vi "Process Mouse Up.vi"(0 "Listbox":refnum<vi>, 1 "Ring":refnum<vi>, 5 "State in":T1, 7 "Coords":T6, 11 "error in (no error)":errorcluster) -> (6 "State out":T1, 8 "state changed":bool, 15 "error out":errorcluster)   [LabVIEW 2020, in "KTable.xctl"]
uses:
  KTable.xctl
  <vilib>/Utility/miscctls.llb/LVPoint32TypeDef.ctl
  State.ctl
  ColumnSpec.ctl
  ColumnType.ctl
  Table Properties.ctl
  Events.ctl
  Event Data.ctl
  Event Type.ctl
  Array Manipulation VIs/Array-Dimensions (2D string).vi
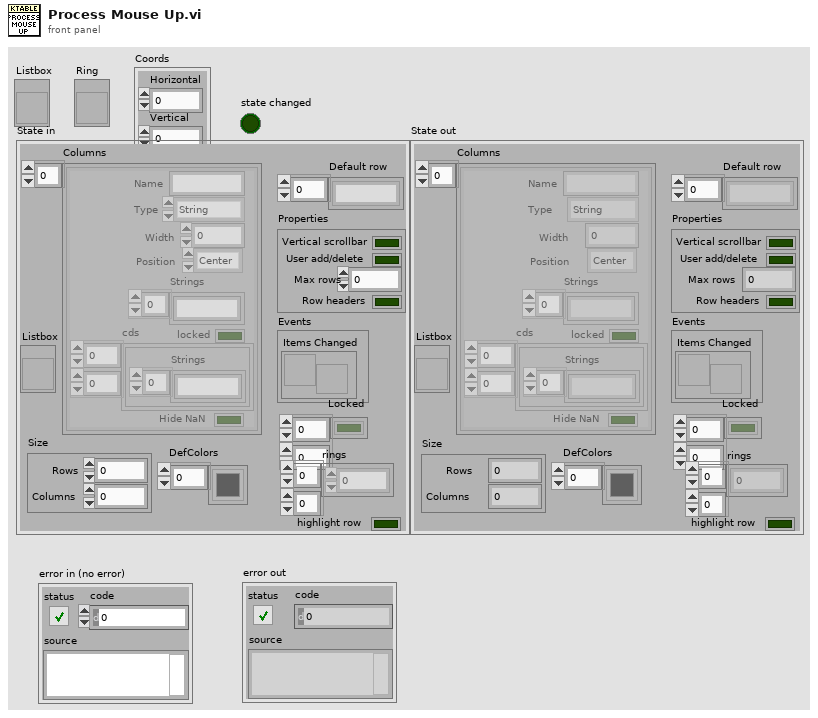
[diagram p1: front panel]
types:
  T1 = typedef "KTable.xctl/State.ctl" = cluster{"Columns":T2[], "Listbox":refnum<vi>, "Default row":string[], "Properties":T4, "Events":T5, "Locked":bool[][], "Size":cluster{"Rows":i32, "Columns":i32}, "rings":i32[][], "DefColors":u32[], "highlight row":bool}
  T2 = typedef "KTable.xctl/ColumnSpec.ctl" = cluster{"Name":string, "Type":T3, "Width":i32, "Strings":string[], "Position":enum16{"Left", "Center", "Right"}, "locked":bool, "cds":cluster{"Strings":string[]}[][], "Hide NaN":bool}
  T3 = typedef "KTable.xctl/ColumnType.ctl" = enum16{"String", "Enum", "Int", "Double", "Boolean", "Ring", "Formula", "Color"}
  T4 = typedef "KTable.xctl/Table Properties.ctl" = cluster{"Vertical scrollbar":bool, "User add/delete":bool, "Max rows":i32, "Row headers":bool}
  T5 = typedef "KTable.xctl/Events.ctl" = cluster{"Items Changed":refnum<user-event>}
  T6 = typedef "LVPoint32TypeDef.ctl" = cluster{"Horizontal":i32, "Vertical":i32}
  T7 = typedef "LVRowAndColumnTypeDef.ctl" = cluster{"Row":i32, "Column":i32}
  T8 = typedef "LVPositionTypeDef.ctl" = cluster{"Left":i32, "Top":i32}
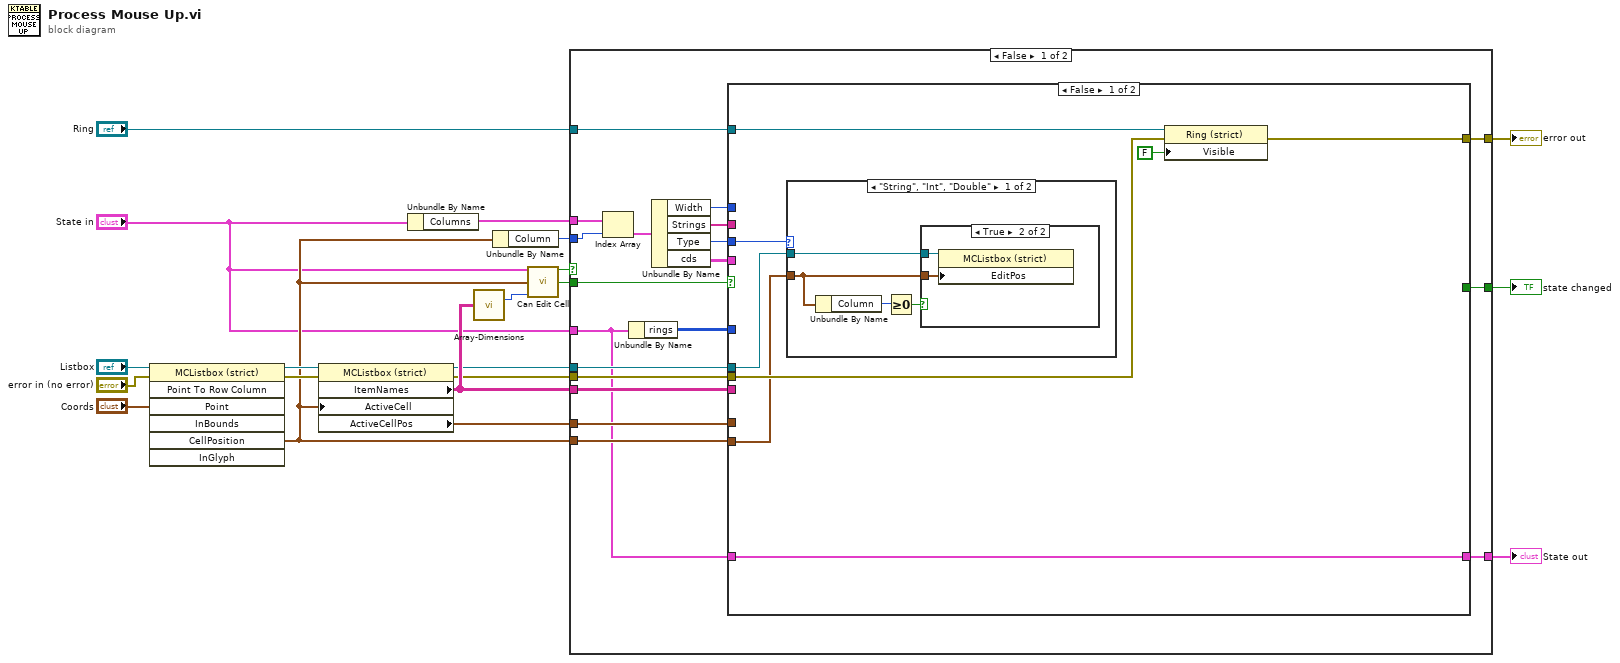
[diagram p0: block diagram]
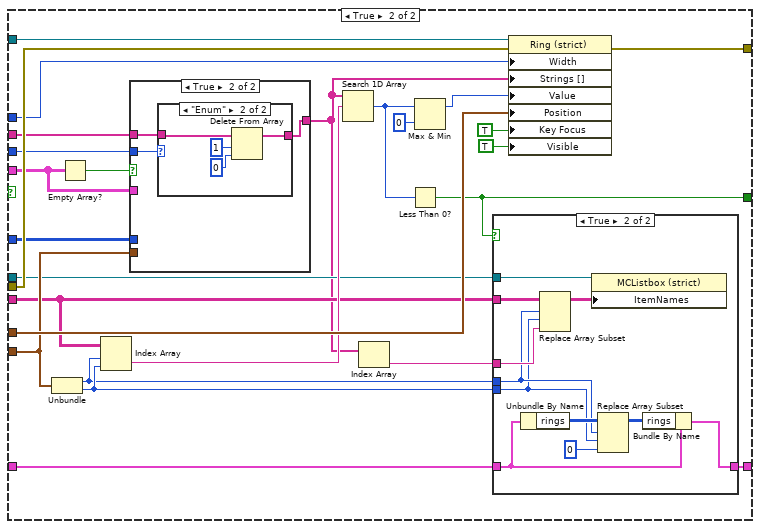
[diagram p4: hidden frame]
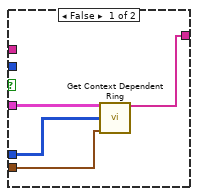
[diagram p6: hidden frame]
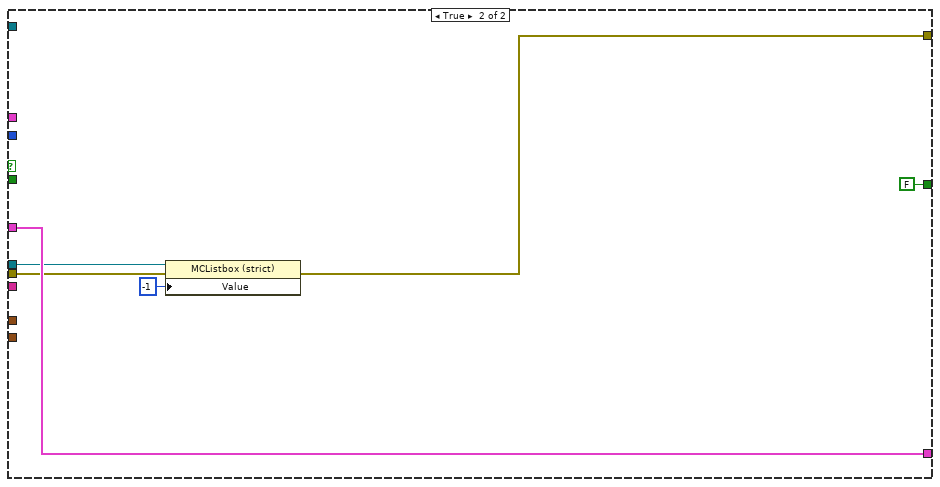
[diagram p8: hidden frame]
diagram:
  n1 = invoke on="Invoke Node" class="MCListbox (strict)" method="Point To Row Column"(reference="Listbox", error in="error in (no error)", "Point"="Coords") -> (reference out=w17:refnum<vi>, error out=w16:errorcluster, "CellPosition"=w10:T7)  [unwired: 4 in, 4 out]
  n2 = property class="MCListbox (strict)"(reference=w17, error in=w16, "ActiveCell"=w10) -> (reference out=w6:refnum<vi>, error out=w12:errorcluster, "ItemNames"=w13:string[][], "ActiveCellPos"=w14:T8)
  n3 = Unbundle By Name("State in") -> ("Columns"=w8:T2[])
  n4 = call-poly "Array-Dimensions.vi"("2D Array"=w13) -> ("# rows"=w9:i32)  [unwired: 13 in, 1 out]
  n5 = Unbundle By Name(w10) -> ("Column"=w7:i32)
  n6 = call "Can Edit Cell.vi"("State"="State in", "Cell"=w10, "NumRows"=w9) -> ("locked"=w1:bool, "can edit?"=w2:bool)  [unwired: 11 in]
  n7 = case shown="False" w1 {
    tunnel: "Ring" -> [w38 _]
    tunnel: w14 -> [w37 _]
    tunnel: w13 -> [w35 _]
    tunnel: w12 -> [w34 w106]
    tunnel: [w33 w105] -> w11
    tunnel: w10 -> [w30 _]
    tunnel: w2 -> [w29 _]
    tunnel: w8 -> [w27 _]
    tunnel: w7 -> [w26 _]
    tunnel: w6 -> [w24 w107]
    tunnel: "State in" -> [w23 w108]
    tunnel: [w22 w108] -> w4
    tunnel: [w21 FALSE] -> w3
    frame False {
      n8 = Index Array(array=w27, index=w26) -> (element=w39:T2)
      n9 = Unbundle By Name(w23) -> ("rings"=w25:i32[][])
      n10 = Unbundle By Name(w39) -> ("Width"=w32:i32, "Strings"=w36:string[], "Type"=w31:T3, "cds"=w28:cluster{"Strings":string[]}[][])
      n11 = case shown="False" w29 {
        tunnel: w38 -> [w46 w77]
        tunnel: w37 -> [_ w75]
        tunnel: w36 -> [_ w69]
        tunnel: w35 -> [_ w62]
        tunnel: w34 -> [w45 w74]
        tunnel: [w44 w73] -> w33
        tunnel: w32 -> [_ w72]
        tunnel: w30 -> [w40 w64]
        tunnel: w31 -> [w42 w68]
        tunnel: w28 -> [_ w65]
        tunnel: w25 -> [_ w66]
        tunnel: w24 -> [w41 w59]
        tunnel: w23 -> [w43 w56]
        tunnel: [w43 w55] -> w22
        tunnel: [_ w54] -> w21
        frame False {
          n12 = case shown="\"String\", \"Int\", \"Double\"" w42 {
            tunnel: w41 -> [w51 _]
            tunnel: w40 -> [w50 _]
            frame "String", "Int", "Double" {
              n13 = Unbundle By Name(w50) -> ("Column"=w49:i32)
              n14 = Greater Or Equal To 0?(x=w49) -> (x >= 0?=w48:bool)
              n15 = case shown="True" w48 {
                tunnel: w51 -> [_ w53]
                tunnel: w50 -> [_ w52]
                frame False {
                }
                frame True {
                  n16 = property class="MCListbox (strict)"(reference=w53, "EditPos"=w52) -> ()  [unwired: 1 in, 2 out]
                }
              }
            }
            frame "Enum", Default {
            }
          }
          n17 = property on="Property Node" class="Ring (strict)"(reference=w46, error in=w45, "Visible"=FALSE) -> (error out=w44:errorcluster)  [unwired: 1 out]
        }
        frame True {
          n18 = Unbundle(w64) -> ("Row"=w60:i32, "Column"=w61:i32)
          n19 = Empty Array?(array=w65) -> (empty?=w67:bool)
          n20 = Index Array(array=w62, index (row)=w60, index (col)=w61) -> (element=w70:string)
          n21 = case shown="True" w67 {
            tunnel: w69 -> [_ w98]
            tunnel: w68 -> [_ w97]
            tunnel: [w95 w96] -> w58
            tunnel: w66 -> [w93 _]
            tunnel: w65 -> [w94 _]
            tunnel: w64 -> [w92 _]
            frame False {
              n22 = call "Get Context Dependent Ring.vi"("cds"=w94, "rings"=w93, "Cell Position"=w92) -> ("Strings"=w95:string[])  [unwired: 12 in]
            }
            frame True {
              n23 = case shown="\"Enum\"" w97 {
                tunnel: w98 -> [w99 w103]
                tunnel: [w99 w102] -> w96
                frame "String", Default {
                }
                frame "Enum" {
                  n24 = Delete From Array(array=w103, length=1, index=0) -> (array with subset deleted=w102:string[])  [unwired: 1 out]
                }
              }
            }
          }
          n25 = Search 1D Array(1D array=w58, element=w70) -> (index of element=w63:i32)  [unwired: 1 in]
          n26 = Index Array(array=w58) -> (element=w57:string)  [unwired: 1 in]
          n27 = Less Than 0?(x=w63) -> (x < 0?=w54:bool)
          n28 = Max & Min(x=w63, y=0) -> (max(x,y)=w71:i32)  [unwired: 1 out]
          n29 = case shown="True" w54 {
            tunnel: w62 -> [_ w91]
            tunnel: w61 -> [_ w82]
            tunnel: w60 -> [_ w83]
            tunnel: w59 -> [_ w90]
            tunnel: w57 -> [_ w88]
            tunnel: w56 -> [w80 w85]
            tunnel: [w80 w84] -> w55
            frame False {
            }
            frame True {
              n30 = Unbundle By Name(w85) -> ("rings"=w87:i32[][])
              n31 = Replace Array Subset(array=w91, new element=w88, index (row)=w83, index (col)=w82) -> (w89:string[][])
              n32 = property class="MCListbox (strict)"(reference=w90, "ItemNames"=w89) -> ()  [unwired: 1 in, 2 out]
              n33 = Replace Array Subset(array=w87, new element=0 ("new element/subarray"), index (row)=w83, index (col)=w82) -> (w86:i32[][])
              n34 = Bundle By Name(cluster=w85, "rings"=w86) -> (w84:T1)
            }
          }
          n35 = property on="Property Node" class="Ring (strict)"(reference=w77, error in=w74, "Width"=w72, "Strings []"=w58, "Value"=w71, "Position"=w75, "Key Focus"=TRUE, "Visible"=TRUE) -> (error out=w73:errorcluster)  [unwired: 1 out]
        }
      }
    }
    frame True {
      n36 = property class="MCListbox (strict)"(reference=w107, error in=w106, "Value"=-1) -> (error out=w105:errorcluster)  [unwired: 1 out]
    }
  }
  "error out" <- w11
  "state changed" <- w3
  "State out" <- w4
